vi "GrabImage.vi"() -> ()   [LabVIEW 2014]
uses:
  4.Other/header ctl/Offset.ctl
  4.Other/header ctl/file number.ctl
  <vilib>/vision/Image Controls.llb/IMAQ Image.ctl
  <vilib>/userdefined/High Color/IMAQdx.ctl
  4.Other/header ctl/Header file data.ctl
  4.Other/header ctl/Offset table.ctl
  <vilib>/Analysis/baseanly.llb/Mean (DBL).vi
  <vilib>/vision/driver/NI_Vision_Acquisition_Software.lvlib
  <resource>/objmgr/imaqdx.rc
  <vilib>/Analysis/NI_AALBase.lvlib
panel:
  out "Saved Frame":u32
  out "avg. fps (Hz)":dbl
  out "acquire time array (ms)":u32[](array[numeric])
  out "frame acquired":i32
  out "Offset array":cluster{"offset":T1, "file number":T2}[](array[cluster])
  out "resized TTB":u32[](array[numeric])
  out "True acquired frame":u32
  in  "Set Gain?":bool
  in  "acquisition time (ms)":u32=30
  out "fps (Hz)":dbl
  out "TTB array (ms)\ntime axis (ms)":u32[](array[numeric])
  out "Write to file num":u32
  out "Glimpse refnum Array":refnum<file>[](array[refnum])
  in  "T = Stop Record":bool
  in  "T = Record Sequence":bool
  out "Finish Save?":bool
  out "Pixel depth":i16
  out "Path String Array":string[](array[string])
  in  "Tab Control":enum32{"Set Parameters", "Image Player"}(tab)
  in  "Set Record Frame#":u32=30000
  out "Width":i32
  out "Height":i32
  in  "Data type":enum16{"U8", "I16"}(ring)
  in  "Select a Folder":path
  out "size of one frame (byte)":u32
  out "Frame# of one .Glimpse \n(2Gb)":u32
  out "Estimated total file size (byte, b)":u32
  out "Estimated total file size (Kb)":dbl
  out "image in Queue":i32(slide) min=0 max=180 step=30 scale=0.18..200.0
  in  "Set Width":dbl=1120.0
  in  "Set Height":dbl=630.0
  out "pixel# of a image":i32
  out "Estimated a file size (byte, b)":u32
  out "Image Display":T3(plugin-control)
  # "width : max 1920"
  # "height max : 1200"
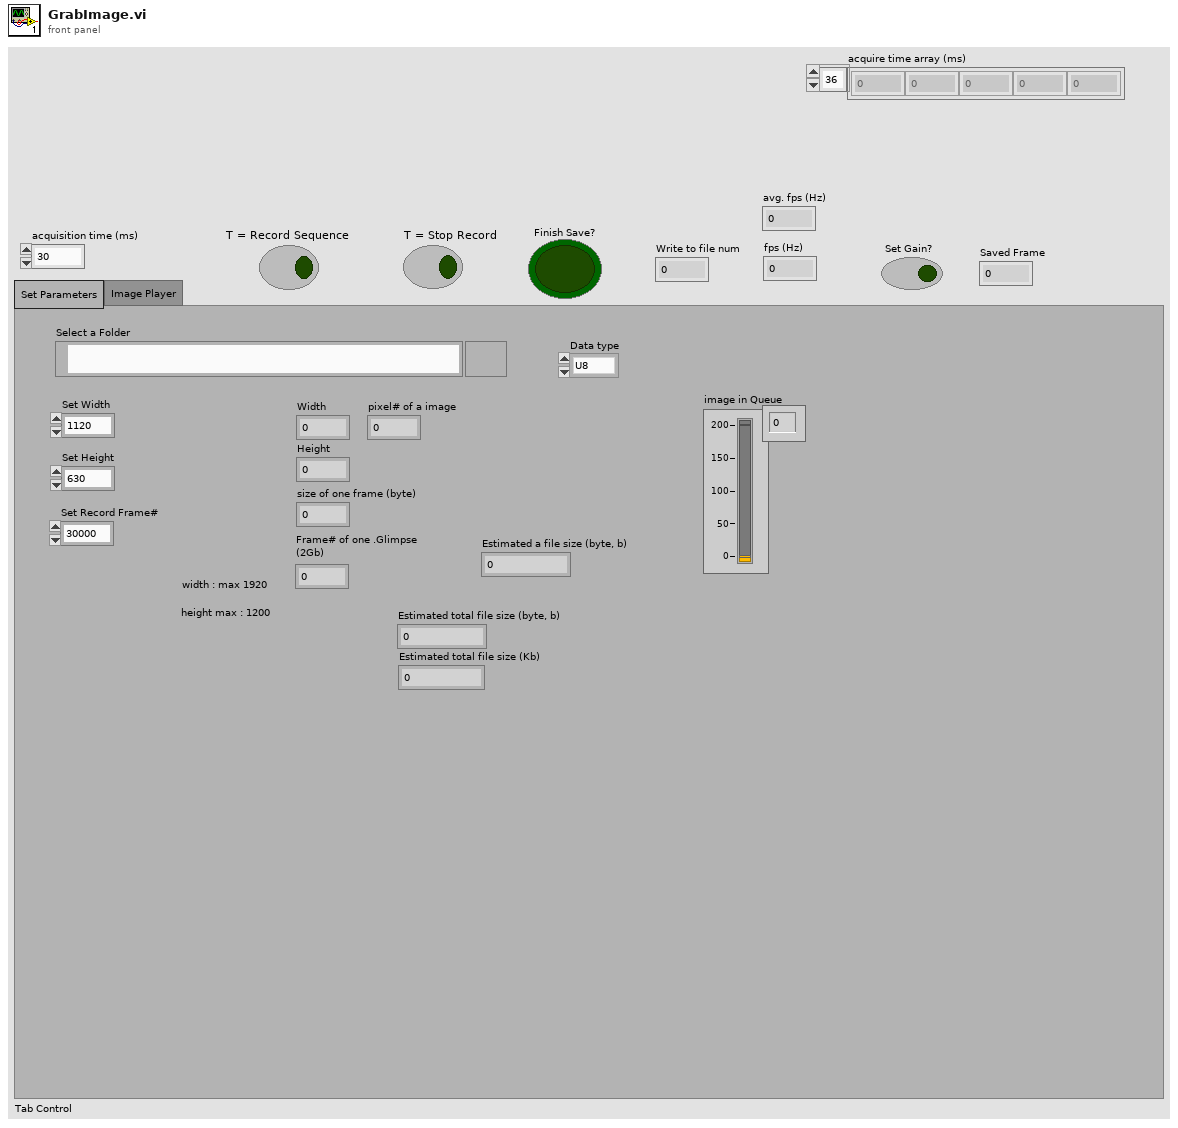
[diagram p1: front panel]
types:
  T1 = typedef "Offset.ctl" = i32
  T2 = typedef "file number.ctl" = u8
  T3 = typedef "IMAQ Image.ctl" = refnum<image>
  T4 = typedef "IMAQdx.ctl" = refnum<k21>
  T5 = typedef "Image Type" = u32
  T6 = cluster{"Grab Image":T3, "max queue size (-1, unlimited)":u32}
  T7 = enum16{"open", "replace", "create", "open or create", "replace or create", "replace or create with confirmation"}
  T8 = typedef "Header file data.ctl" = cluster{"Frames Acquired":u32, "Region width":i32, "Region height":i32, "Element 0 of TTB":u32, "time of 1st frame, \nsec since 1/1/04":dbl, "TTB Array (ms)":u32[], "Offsets Array":T9, "Pixel depth":u32}
  T9 = typedef "Offset table.ctl" = cluster{"offset":T1, "file number":T2}[]
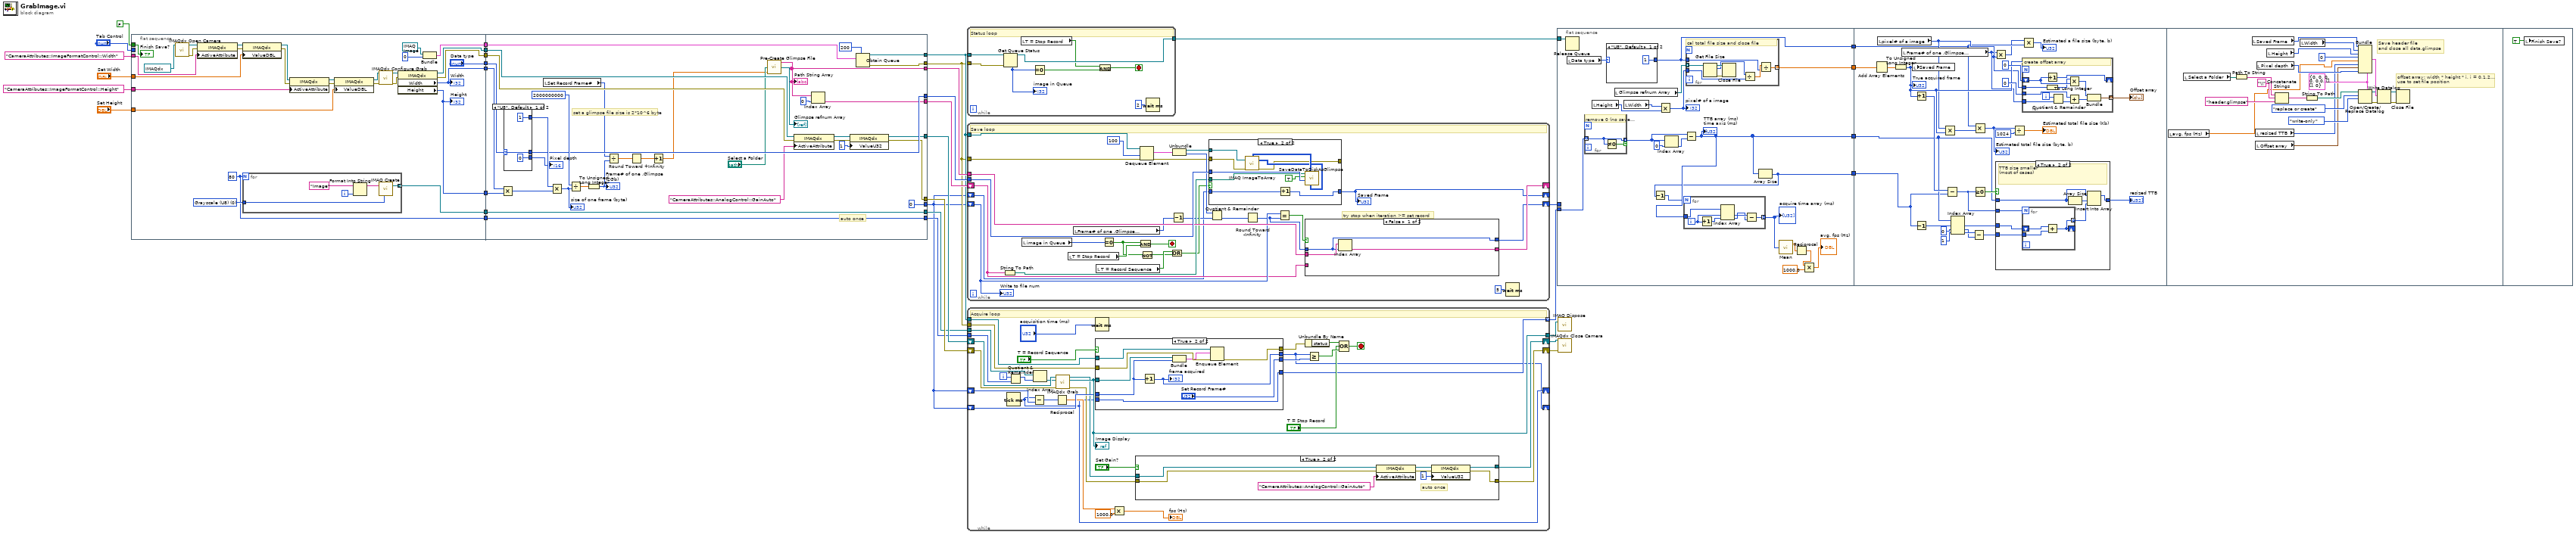
[diagram p0: block diagram]
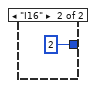
[diagram p2: hidden frame]
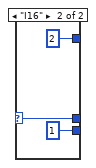
[diagram p4: hidden frame]
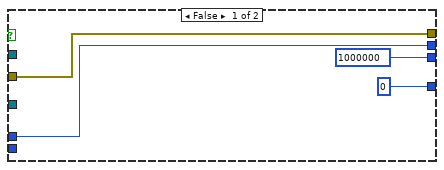
[diagram p8: hidden frame]
diagram:
  n1 = flat-sequence {
    tunnel: [w54] -> w31
    tunnel: [w53] -> w30
    tunnel: [w63] -> w27
    tunnel: [w62] -> w26
    tunnel: ["Data type"] -> w24
    tunnel: [w58] -> w22
    tunnel: [w51] -> w19
    tunnel: [w50] -> w17
    tunnel: "Tab Control" -> [_]
    tunnel: FALSE ("Finish Save?") -> [w39]
    tunnel: "CameraAttributes::ImageFormatControl::Width" ("Active Item:Tag") -> [w38]
    tunnel: "CameraAttributes::ImageFormatControl::Height" ("Active Item:Tag") -> [w37]
    tunnel: "Set Width" -> [w36]
    tunnel: "Set Height" -> [w35]
    tunnel: [w78] -> w28
    tunnel: w31 -> [w81]
    tunnel: [w77] -> w29
    tunnel: w30 -> [w79]
    tunnel: w27 -> [w103]
    tunnel: w26 -> [w102]
    tunnel: w24 -> [w96]
    tunnel: [w95] -> w23
    tunnel: w22 -> [w89]
    tunnel: [w94] -> w18
    tunnel: w19 -> [w94]
    tunnel: [w93] -> w16
    tunnel: w17 -> [w93]
    tunnel: [w75] -> w14
    tunnel: [0] -> w7
    tunnel: [w90] -> w10
    tunnel: [w88] -> w9
    tunnel: [w87] -> w8
    frame #0 {
      w50 = 80 ("# Of Buffers")
      w52 = T5 0 items=["Grayscale (U8)", "Grayscale (I16)", "Grayscale (SGL)", "Complex (CSG)", "RGB (U32)", "HSL (U32)", "RGB (U64)", "Grayscale (U16)"] ("Image Type")
      n2 = call <vilib>:"IMAQdx Open Camera.vi"("Session In"=T4 "cam2") -> ("error out"=w48:errorcluster, "Session Out"=w49:T4)  [unwired: 9 in]
      n3 = property class="IMAQdx"(reference=w49, error in=w48, "ActiveAttribute"=w38) -> (reference out=w47:T4, error out=w46:errorcluster)
      n4 = property class="IMAQdx"(reference=w47, error in=w46, "ValueDBL"=w36) -> (reference out=w45:T4, error out=w42:errorcluster)
      n5 = for {
        N: w50 -> [_]
        tunnel: [w68] -> w51 mode=indexing
        tunnel: w52 -> [w64]
        i -> [w67]
        n6 = Format Into String(initial string="Image" ("Image Name"), w67) -> (resulting string=w65:string)  [unwired: 2 in, 1 out]
        n7 = call "IMAQ Create"("Image Name"=w65, "Image Type"=w64) -> ("New Image"=w68:T3)  [unwired: 3 in, 1 out]
      }
      n8 = property class="IMAQdx"(reference=w45, error in=w42, "ActiveAttribute"=w37) -> (reference out=w44:T4, error out=w41:errorcluster)
      n9 = property class="IMAQdx"(reference=w44, error in=w41, "ValueDBL"=w35) -> (reference out=w43:T4, error out=w40:errorcluster)
      n10 = call <vilib>:"IMAQdx Configure Grab.vi"("error in"=w40, "Session In"=w43) -> ("error out"=w55:errorcluster, "Session Out"=w56:T4)  [unwired: 8 out]
      n11 = property class="IMAQdx"(reference=w56, error in=w55) -> (reference out=w54:T4, error out=w53:errorcluster, "Width"=w63:u32, "Height"=w62:u32)
      "Width" <- w63
      "Height" <- w62
      n12 = Bundle("Grab Image"=T3 refnum, "max queue size (-1, unlimited)"=u32 0) -> (w58:T6)  [unwired: 1 in]
      "Finish Save?" <- w39
    }
    frame #1 {
      # "auto once"
      # "set a glimpse file size is 2*10^6 byte"
      n13 = Multiply(x=w103, y=w102) -> (x*y=w101:u32)
      n14 = case shown="\"U8\", Default" w96 {
        selector: w96 -> [w105 w108]
        tunnel: [1 2] -> w100
        tunnel: [w105 w108] -> w95
        tunnel: [i16 0 i16 1] -> w85
        frame "U8", Default {
        }
        frame "I16" {
        }
      }
      "Pixel depth" <- w85
      n15 = local read "Set Record Frame#"() -> (w73:u32)
      n16 = Multiply(x=w100, y=w101) -> (x*y=w98:u32)
      "size of one frame (byte)" <- w98
      n17 = Divide(x=2000000000, y=w98) -> (x/y=w97:dbl)
      n18 = To Unsigned Long Integer(number=w97) -> (unsigned 32bit integer=w72:u32)
      "Frame# of one .Glimpse \n(2Gb)" <- w72
      n19 = Divide(x=w73, y=w72) -> (x/y=w71:dbl)
      n20 = Round Toward +Infinity(x=w71) -> (ceil(x): smallest int >= x=w70:dbl)
      n21 = Increment(x=w70) -> (x+1=w69:dbl)
      n22 = call "Pre-Create Glimpse File.vi"("pre-created file #"=w69, "Select a Folder"="Select a Folder") -> ("refnum Array"=→"Glimpse refnum Array":refnum<file>[], "Path String Array"=w75:string[])  [unwired: 2 in]
      "Path String Array" <- w75
      n23 = property class="IMAQdx"(reference=w81, error in=w79, "ActiveAttribute"="CameraAttributes::AnalogControl::GainAuto") -> (reference out=w84:T4, error out=w83:errorcluster)
      n24 = Index Array(array=w75, index=0) -> (element=w90:string)
      n25 = property class="IMAQdx"(reference=w84, error in=w83, "ValueU32"=u32 1) -> (reference out=w78:T4, error out=w77:errorcluster)
      n26 = Obtain Queue(max queue size (-1, unlimited)=200, element data type=w89) -> (queue out=w88:refnum<queue>, error out=w87:errorcluster)  [unwired: 3 in, 1 out]
    }
  }
  n27 = while {
    tunnel: w9 -> [w117]
    tunnel: [w116] -> w20
    tunnel: w8 -> [w115]
    stop <- w110 stop-if-true
    # "Status loop"
    n28 = Get Queue Status(queue=w117, error in (no error)=w115) -> (queue out=w116:refnum<queue>, # elements in queue=w113:i32)  [unwired: 1 in, 6 out]
    "image in Queue" <- w113
    n29 = local read "T = Stop Record"() -> (w111:bool)
    n30 = Equal To 0?(x=w113) -> (x = 0?=w114:bool)
    n31 = And(x=w111, y=w114) -> (x .and. y?=w110:bool)
    n32 = Wait (ms)(milliseconds to wait=u32 2) -> ()  [unwired: 1 out]
  }
  n33 = while {
    tunnel: w9 -> [w146]
    tunnel: w8 -> [w145]
    tunnel: w23 -> [w144]
    shift-right: [w133] -> w21
    shift-left: w7 -> [w138]
    shift-right: [w137] -> _
    shift-left: w10 -> [w135]
    tunnel: w14 -> [w139]
    shift-right: [w118] -> _
    shift-left: w7 -> [w119]
    stop <- w122 stop-if-true
    # "try stop when iteration >= set record"
    # "Save loop"
    n34 = String To Path(string=w135) -> (path=w136:path)
    n35 = local read "image in Queue"() -> (w128:i32)
    n36 = local read "T = Stop Record"() -> (w130:bool)
    n37 = local read "Frame# of one .Glimpse \n(2Gb)"() -> (w120:u32)
    n38 = local read "T = Record Sequence"() -> (w127:bool)
    n39 = Equal To 0?(x=w128) -> (x = 0?=w125:bool)
    n40 = And(x=w125, y=w130) -> (x .and. y?=w122:bool)
    n41 = Dequeue Element(queue=w146, timeout in ms (-1)=100, error in (no error)=w145) -> (element=w143:T6, error out=w129:errorcluster)  [unwired: 2 out]
    n42 = Not(x=w125) -> (.not. x?=w126:bool)
    n43 = Or(x=w127, y=w126) -> (x .or. y?=w124:bool)
    n44 = Decrement(x=w120) -> (x-1=w121:u32)
    n45 = Unbundle(w143) -> ("Grab Image"=w132:T3, "max queue size (-1, unlimited)"=w142:u32)
    n46 = case shown="True" w124 {
      tunnel: w144 -> [_ w158]
      tunnel: w136 -> [_ w157]
      tunnel: w132 -> [_ w153]
      tunnel: w129 -> [w148 w152]
      tunnel: [w148 w151] -> _
      tunnel: w119 -> [w147 w150]
      tunnel: [w147 w149] -> w118
      frame False {
      }
      frame True {
        n47 = call "IMAQ ImageToArray"("error in (no error)"=w152, "Image"=w153) -> ("error out"=w151:errorcluster, "Image Pixels (U8)"=w155:u8[][], "Image Pixels (I16)"=w154:i16[][])  [unwired: 2 in, 2 out]
        n48 = Increment(x=w150) -> (x+1=w149:i32)
        n49 = call "SaveDataToDiskAsGlimpse.vi"("Read or Write Path"=w157, "Array (U8)"=w155, "T = AddNewData\nF = if exist, OverWrite or CreateNew"=TRUE ("T = AddNewData\nF = if exist, OverWrite or CreateNew"), "Data type"=w158, "Array (I16)"=w154) -> ()  [unwired: 3 in, 1 out]
      }
    }
    "Saved Frame" <- w118
    n50 = Quotient & Remainder(x=w142, y=w121) -> (floor(x/y)=w141:u32)  [unwired: 1 out]
    n51 = Round Toward -Infinity(1:w141) -> (0:w134:u32)
    n52 = Equal?(x=w138, y=w134) -> (x = y?=w140:bool)
    n53 = case shown="False" w140 {
      tunnel: w139 -> [w161 _]
      tunnel: w134 -> [w159 w162]
      tunnel: [w160 w163] -> w137
      tunnel: w135 -> [_ w163]
      tunnel: [w159 w162] -> w133
      frame False {
        n54 = Index Array(array=w161, index=w159) -> (element=w160:string)
      }
      frame True {
        # "not to exceed a set-glimpse size"
      }
    }
    n55 = Wait (ms)(milliseconds to wait=u32 5) -> ()  [unwired: 1 out]
    "Write to file num" <- w138
  }
  n56 = while {
    tunnel: [w188] -> w32
    tunnel: w9 -> [w192]
    shift-right: [w165] -> _
    shift-left: w7 -> [w187]
    tunnel: w8 -> [w186]
    shift-right: [w167] -> _
    shift-left: w7 -> [w185]
    tunnel: w18 -> [w178]
    tunnel: w16 -> [w176]
    tunnel: [w166] -> w15 mode=indexing
    shift-right: [w168] -> w34
    shift-left: w28 -> [w195]
    shift-right: [w169] -> w33
    shift-left: w29 -> [w194]
    i -> [w179]
    stop <- w173 stop-if-true
    # "Acquire loop"
    n57 = Tick Count (ms)() -> (millisecond timer value=w167:u32)
    n58 = Quotient & Remainder(x=w179, y=w176) -> (x-y*floor(x/y)=w180:i32)  [unwired: 1 out]
    n59 = Subtract(x=w167, y=w185) -> (x-y=w184:u32)
    n60 = Index Array(array=w178, index=w180) -> (element=w177:T3)
    n61 = Reciprocal(x=w184) -> (1/x=w183:dbl)
    n62 = call <vilib>:"IMAQdx Grab.vi"("error in"=w194, "Image In"=w177, "Session In"=w195) -> ("error out"=w170:errorcluster, "Image Out"=w188:T3, "Session Out"=w171:T4)  [unwired: 1 in, 5 out]
    "Image Display" <- w188
    n63 = Wait (ms)(milliseconds to wait="acquisition time (ms)") -> ()  [unwired: 1 out]
    n64 = case shown="True" "T = Record Sequence" {
      tunnel: w192 -> [_ w218]
      tunnel: w188 -> [_ w215]
      tunnel: w186 -> [w209 w217]
      tunnel: [w209 w216] -> w191
      tunnel: w187 -> [w208 w214]
      tunnel: [w208 w213] -> w165
      tunnel: [u32 1000000 ("Set Record Frame#") "Set Record Frame#"] -> w174
      tunnel: [u32 0 ("millisecond timer value") w210] -> w166
      tunnel: w167 -> [_ w210]
      frame False {
      }
      frame True {
        n65 = Increment(x=w214) -> (x+1=w213:i32)
        "frame acquired" <- w213
        n66 = Bundle("Image Out"=w215, w214) -> (w212:cluster{"Image Out":T3, i32})  [unwired: 1 in]
        n67 = Enqueue Element(queue=w218, element=w212, error in (no error)=w217) -> (error out=w216:errorcluster)  [unwired: 1 in, 2 out]
      }
    }
    n68 = Multiply(x=w183, y=1000.0) -> (x*y=→"fps (Hz)":dbl)
    n69 = case shown="True" "Set Gain?" {
      tunnel: w171 -> [w197 w204]
      tunnel: w170 -> [w196 w203]
      tunnel: [w196 w198] -> w169
      tunnel: [w197 w199] -> w168
      frame False {
      }
      frame True {
        # "auto once"
        n70 = property class="IMAQdx"(reference=w204, error in=w203, "ActiveAttribute"="CameraAttributes::AnalogControl::GainAuto") -> (reference out=w202:T4, error out=w201:errorcluster)
        n71 = property class="IMAQdx"(reference=w202, error in=w201, "ValueU32"=u32 1) -> (reference out=w199:T4, error out=w198:errorcluster)
      }
    }
    n72 = Unbundle By Name(w191) -> ("status"=w193:bool)
    n73 = Greater Or Equal?(x=w165, y=w174) -> (x >= y?=w190:bool)
    n74 = Compound Arithmetic op=OR(w193, "T = Stop Record", w190) -> (w173:bool)
  }
  n75 = flat-sequence {
    tunnel: w21 -> [_]
    tunnel: w15 -> [w228]
    tunnel: w20 -> [w237]
    tunnel: [w230] -> w13
    tunnel: [w226] -> w12
    tunnel: [w229] -> w11
    tunnel: [w225] -> w1
    tunnel: w13 -> [w278]
    tunnel: w12 -> [w266]
    tunnel: w11 -> [w262]
    tunnel: w1 -> [w257]
    frame #0 {
      n76 = Release Queue(queue=w237) -> ()  [unwired: 1 in, 4 out]
      n77 = local read "Data type"() -> (w232:enum16{"U8", "I16"})
      n78 = for {
        tunnel: w228 -> [w246] mode=indexing
        tunnel: [w246] -> w227 mode=indexing if=w245
        # "remove 0 (no save frame)"
        n79 = Not Equal To 0?(x=w246) -> (x != 0?=w245:bool)
      }
      n80 = local read "Height"() -> (w235:i32)
      n81 = case shown="\"U8\", Default" w232 {
        tunnel: [1 2] -> w229
        frame "U8", Default {
        }
        frame "I16" {
        }
      }
      n82 = local read "Glimpse refnum Array"() -> (w238:refnum<file>[])
      n83 = local read "Width"() -> (w236:i32)
      n84 = Multiply(x=w236, y=w235) -> (x*y=w231:i32)
      "pixel# of a image" <- w231
      n85 = Index Array(array=w227, index=0) -> (element=w234:u32)
      n86 = Subtract(x=w227, y=w234) -> (x-y=w226:u32[])
      "TTB array (ms)\ntime axis (ms)" <- w226
      n87 = for {
        tunnel: w238 -> [w256] mode=indexing
        tunnel: w231 -> [w252]
        tunnel: [w249] -> w230 mode=indexing
        tunnel: w229 -> [w250]
        # "cal total file size and close file"
        n88 = Get File Size(file=w256) -> (refnum out=w255:refnum<file>, size (in bytes)=w253:i64, 0:w254:errorcluster)  [unwired: 1 in]
        n89 = Close File(refnum=w255, error in=w254) -> ()  [unwired: 2 out]
        n90 = Divide(x=w253, y=w252) -> (x/y=w251:dbl)
        n91 = Divide(x=w251, y=w250) -> (x/y=w249:dbl)
      }
      n92 = Array Size(array=w226) -> (size(s)=w225:i32)
      n93 = Decrement(x=w225) -> (x-1=w224:i32)
      n94 = for {
        N: w224 -> [_]
        tunnel: w226 -> [w244]
        tunnel: [w239] -> w223 mode=indexing
        i -> [w243]
        n95 = Increment(x=w243) -> (x+1=w242:i32)
        n96 = Index Array(array=w244, index #1=w243, index #2=w242) -> (element #1=w240:u32, element #2=w241:u32)
        n97 = Subtract(x=w241, y=w240) -> (x-y=w239:u32)
      }
      "acquire time array (ms)" <- w223
      n98 = call-poly <vilib>:"Mean.vi"("X"=w223) -> ("mean"=w222:dbl)  [unwired: 1 out]
      n99 = Reciprocal(x=w222) -> (1/x=w221:dbl)
      n100 = Multiply(x=w221, y=1000.0) -> (x*y=→"avg. fps (Hz)":dbl)
    }
    frame #1 {
      n101 = Add Array Elements(numeric array=w278) -> (sum=w277:dbl)
      n102 = local read "pixel# of a image"() -> (w263:i32)
      n103 = To Unsigned Long Integer(number=w277) -> (unsigned 32bit integer=w273:u32)
      "True acquired frame" <- w273
      n104 = local read "Frame# of one .Glimpse \n(2Gb)"() -> (w259:u32)
      n105 = local write "Saved Frame"(w273) -> ()
      n106 = Increment(x=w273) -> (x+1=w271:u32)
      n107 = Decrement(x=w257) -> (x-1=w264:i32)
      n108 = Multiply(x=w263, y=w273) -> (x*y=w272:u32)
      n109 = Subtract(x=w271, y=w257) -> (x-y=w269:u32)
      n110 = Index Array(array=w266, index #1=w264, index #2=0 ("index"), index #3=1 ("index")) -> (element #1=w268:u32, element #2=w283:u32, element #3=w284:u32)
      n111 = Subtract(x=w284, y=w283) -> (x-y=w267:u32)
      n112 = Multiply(x=w262, y=w272) -> (x*y=w274:u32)
      "Estimated total file size (byte, b)" <- w274
      n113 = Greater Or Equal To 0?(x=w269) -> (x >= 0?=w270:bool)
      n114 = Multiply(x=w259, y=w263) -> (x*y=w261:u32)
      n115 = case shown="True" w270 {
        tunnel: w269 -> [_ w292]
        tunnel: w268 -> [_ w291]
        tunnel: w267 -> [_ w290]
        tunnel: w266 -> [w285 w288]
        tunnel: [w285 w287] -> w265
        frame False {
          # "TTB size always >= acquired frame"
        }
        frame True {
          # "TTB size smaller \n(most of cases)"
          n116 = for {
            N: w292 -> [_]
            tunnel: w290 -> [w294]
            shift-right: [w293] -> _
            shift-left: w291 -> [w295]
            tunnel: [w293] -> w289 mode=indexing
            n117 = Add(x=w295, y=w294) -> (x+y=w293:u32)
          }
          n118 = Array Size(array=w288) -> (size(s)=w286:i32)
          n119 = Insert Into Array(array=w288, index=w286, new element=w289) -> (w287:u32[])
        }
      }
      "resized TTB" <- w265
      n120 = Divide(x=w274, y=u32 1024) -> (x/y=→"Estimated total file size (Kb)":dbl)
      n121 = Multiply(x=w261, y=w262) -> (x*y=→"Estimated a file size (byte, b)":u32)
      n122 = for {
        N: w273 -> [_]
        tunnel: w263 -> [w303]
        tunnel: [w306] -> w258 mode=indexing
        shift-right: [w305] -> _
        shift-left: T1 0 ("offset") -> [w304]
        tunnel: T2 0 ("file number") -> [w300]
        tunnel: w259 -> [w298]
        i -> [w297]
        # "create offset array"
        n123 = Increment(x=w304) -> (x+1=w305:T1)
        n124 = To Long Integer(number=w303) -> (32bit integer=w302:i32)
        n125 = Quotient & Remainder(x=w297, y=w298) -> (floor(x/y)=w299:u32)  [unwired: 1 out]
        n126 = Multiply(x=w302, y=w304) -> (x*y=w301:T1)
        n127 = Add(x=w300, y=w299) -> (x+y=w296:u32)
        n128 = Bundle("offset"=w301, w296) -> (w306:cluster{"offset":T1, u32})  [unwired: 1 in]
      }
      "Offset array" <- w258
    }
    frame #2 {
      w323 = T8 {"Frames Acquired"=0, "Region width"=0, "Region height"=0, "Element 0 of TTB"=0, "time of 1st frame, \nsec since 1/1/04"=0.0, "TTB Array (ms)"=[], "Offsets Array"=[], "Pixel depth"=0} ("Header file data")
      # "offset array: width * height * i, i = 0,1,2...\nuse to set file position"
      # "Save header file\nand close all data.glimpse"
      n129 = local read "avg. fps (Hz)"() -> (w307:dbl)
      n130 = local read "Select a Folder"() -> (w317:path)
      n131 = Path To String(path=w317) -> (string=w315:string)
      n132 = local read "Saved Frame"() -> (w318:u32)
      n133 = local read "resized TTB"() -> (w309:u32[])
      n134 = local read "Offset array"() -> (w308:cluster{"offset":T1, "file number":T2}[])
      n135 = local read "Pixel depth"() -> (w322:i16)
      n136 = local read "Height"() -> (w320:i32)
      n137 = Concatenate Strings(w315, "\\" ("string"), "header.glimpse" ("string")) -> (w314:string)
      n138 = local read "Width"() -> (w319:i32)
      n139 = String To Path(string=w314) -> (path=w312:path)
      n140 = Bundle(cluster=w323, "Frames Acquired"=w318, "Region width"=w319, "Region height"=w320, "Element 0 of TTB"=u32 0, "time of 1st frame, \nsec since 1/1/04"=w307, "TTB Array (ms)"=w309, "Offsets Array"=w308, "Pixel depth"=w322) -> (w328:T8)
      n141 = Open/Create/Replace Datalog(5:w323, 9:enum16{"read/write", "read-only", "write-only"}."write-only" ("access (0:read/write)"), 10:T7."replace or create" ("operation (0:open)"), 11:w312) -> (0:w326:errorcluster, 3:w324:refnum<k1>)  [unwired: 1 in, 2 out]
      n142 = Write Datalog(4:w326, 6:w328, 7:w324) -> (0:w327:errorcluster, 3:w325:refnum<k1>)
      n143 = Close File(refnum=w325, error in=w327) -> ()  [unwired: 2 out]
    }
    frame #3 {
      n144 = local write "Finish Save?"(TRUE) -> ()
    }
  }
  n145 = call "IMAQ Dispose"("Image"=w32) -> ()  [unwired: 5 in, 1 out]
  n146 = call <vilib>:"IMAQdx Close Camera.vi"("error in"=w33, "Session In"=w34) -> ()  [unwired: 10 out]
